vi "load_xml_2.vi"(8 "error in":errorcluster, 10 "child node in":refnum<k20>, 11 "HSDIO (in)":refnum<class "HSDIO.lvclass">) -> (0 "error out":errorcluster, 2 "child node out":refnum<k20>, 3 "HSDIO":refnum<class "HSDIO.lvclass">)   [LabVIEW 2013, in "HSDIO.lvclass"]
doc: "Loads HSDIO settings from xml. Expected format:\n\n<EnableHSDIOPulses>%b</EnableHSDIOPulses>\n<ResourceName>%s</ResourceName>\n<ClockRate>%f</ClockRate>\n<unitsPerSecond>%f</unitsPerSecond>\n<HardwareAlignmentQuantum units=\"samples\">%u</HardwareAlignmentQuantum>\n<ArrayOfScriptTriggers columns=\"id, source, type, edge, level\">\n<trigger>%s\\t%s\\t%s\\t%s\\t%s</trigger>\n</ArrayOfScriptTriggers>\n<ChannelsControl columns=\"Description, Active?, Idle State\">\n<channel>%s</channel>\n</ChannelsControl>\n<PulseGenerationScript>%s</PulseGenerationScript>\n<DirectoryToLookForWaveformFiles>%s</DirectoryToLookForWaveformFiles>\n<StartTrigger.WaitForStartTrigger>%b</StartTrigger.WaitForStartTrigger>\n<StartTrigger.source>%s</StartTrigger.source>\n<StartTrigger.edge>%s</StartTrigger.edge>\n\nMTL 2013 Jan 1"
uses:
  HSDIO.lvclass
  HSDIO.lvclass/HSDIO.ctl
  <instrlib>/niHSDIO/niHSDIO.llb/niHSDIO_ctl Trigger Script - trigID Values (Ring).ctl
  <instrlib>/niHSDIO/niHSDIO.llb/niHSDIO_ctl Trigger Source Values (Ring).ctl
  <instrlib>/niHSDIO/niHSDIO.llb/niHSDIO_ctl Trigger DigEdge - Edge Values (Ring).ctl
  <instrlib>/niHSDIO/niHSDIO.llb/niHSDIO_ctl Trigger DigLvl - Level Values (Ring).ctl
  waveform.ctl
  <vilib>/xml/Close Reference(Node).vi
  <resource>/objmgr/DOMUserDefRef.rc
  <vilib>/xml/NI_XML.lvlib
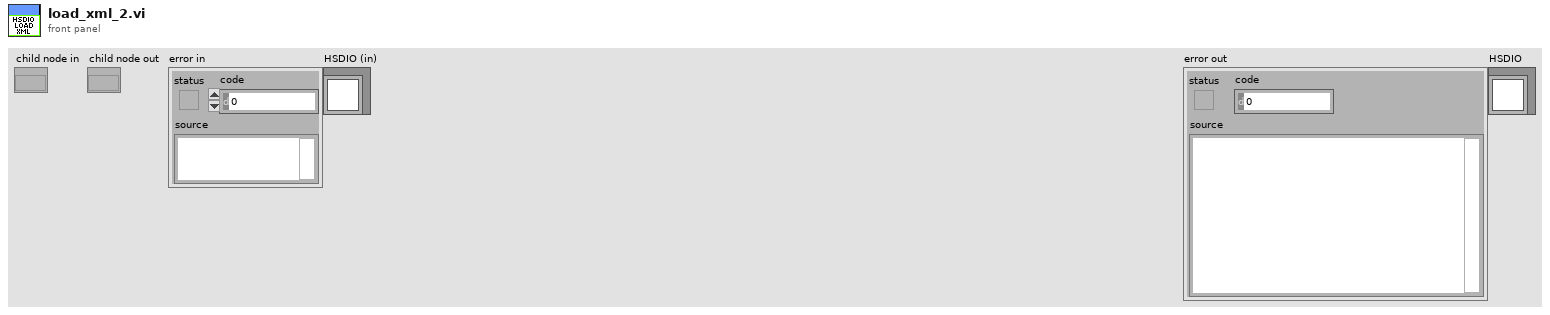
[diagram p1: front panel]
types:
  T1 = typedef "niHSDIO_ctl Trigger Script - trigID Values (Ring).ctl" = string
  T2 = typedef "niHSDIO_ctl Trigger Source Values (Ring).ctl" = string
  T3 = typedef "niHSDIO_ctl Trigger DigEdge - Edge Values (Ring).ctl" = i32
  T4 = typedef "niHSDIO_ctl Trigger DigLvl - Level Values (Ring).ctl" = i32
  T5 = cluster{"trigger id (script trigger 0)":T1, "source (PFI 0)":T2, "Trigger Type":enum32{"Edge", "Level"}, "edge":T3, "level":T4}
  T6 = typedef "HSDIO.lvclass/HSDIO_settings.ctl" = cluster{"Enable HSDIO Pulses":bool, "Resource Name":refnum<k15>, "Clock Rate":dbl, "units/sec (ms=1000)":dbl, "Array of Script Triggers":cluster{"trigger id (script trigger 0)":T1, "source (PFI 0)":T2, "Trigger Type":enum32{"Edge", "Level"}, "edge":T3, "level":T4}[], "Channels Control":string[][], "Pulse Generation Script":string, "Directory to look for waveform files":path, "Start Trigger":cluster{"Wait for start trigger?":bool, "source (PFI 0)":T2, "edge (rising)":T3}, "Hardware alignment quantum\n(in samples)":u16, "Use file script":bool, "Base path for script":path, "filename for script":string, "Inital State":string, "Idle State":string, "Active Channels":string, "Array of Waveforms":T7[]}
  T7 = typedef "HSDIO.lvclass/waveform.ctl" = cluster{"name":string, "transitions":u32[], "states":u8[][]}
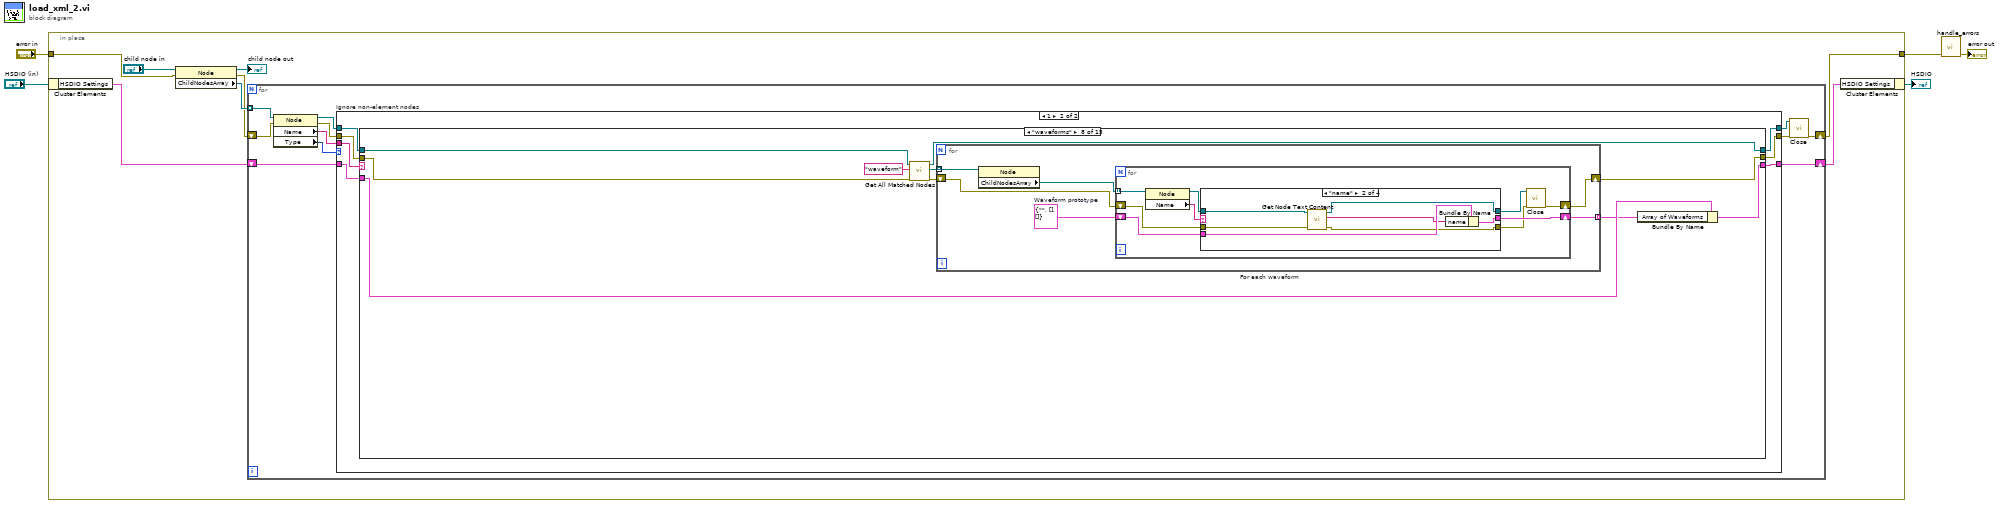
[diagram p0: block diagram]
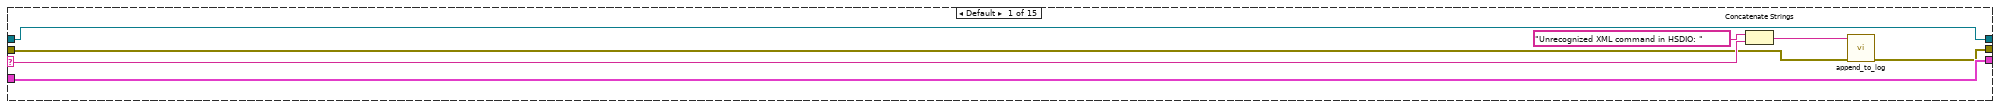
[diagram p3: hidden frame]
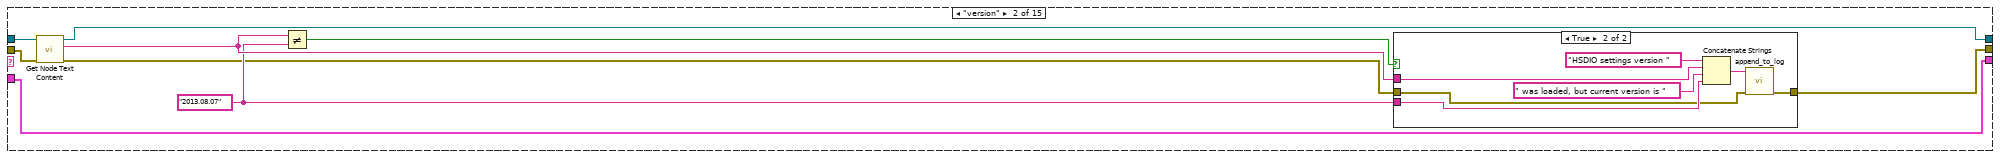
[diagram p4: hidden frame]
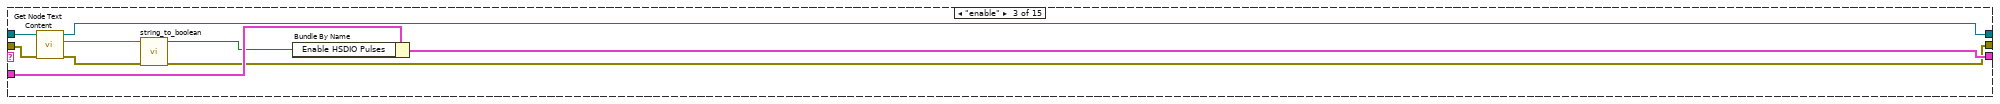
[diagram p6: hidden frame]
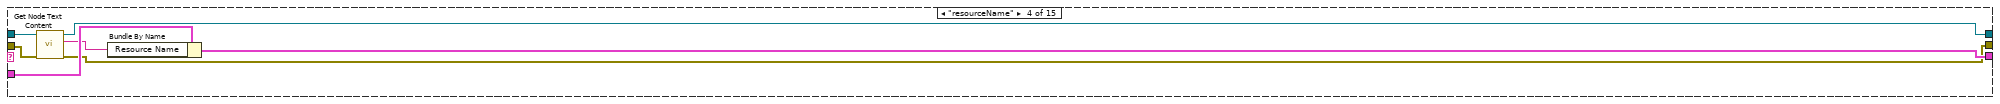
[diagram p7: hidden frame]
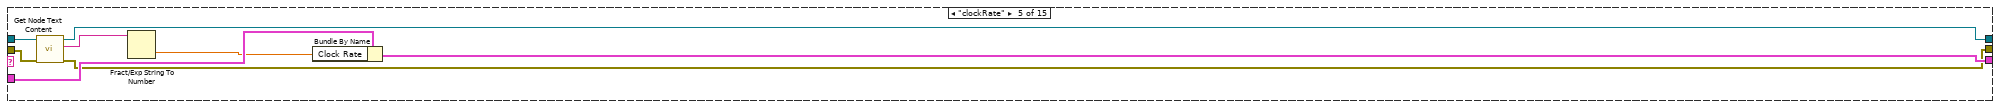
[diagram p8: hidden frame]
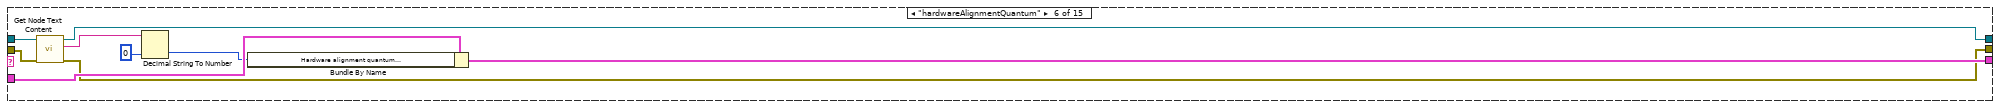
[diagram p9: hidden frame]
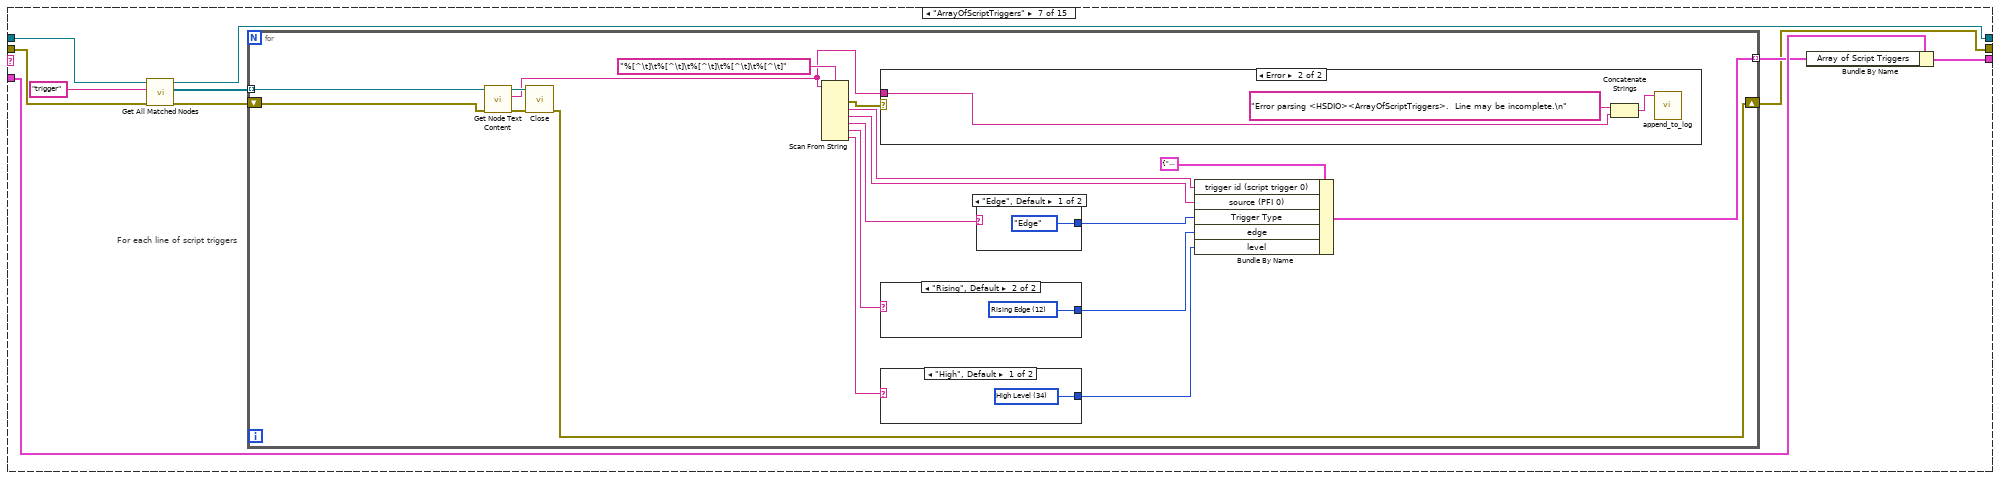
[diagram p10: hidden frame]
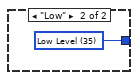
[diagram p11: hidden frame]
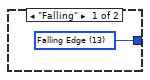
[diagram p12: hidden frame]
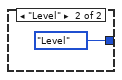
[diagram p13: hidden frame]
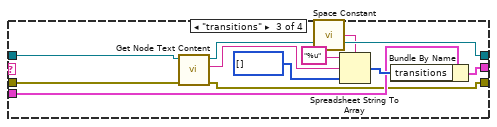
[diagram p16: hidden frame]
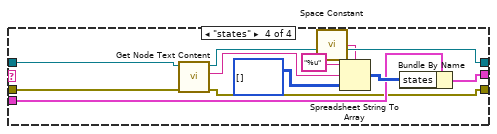
[diagram p17: hidden frame]
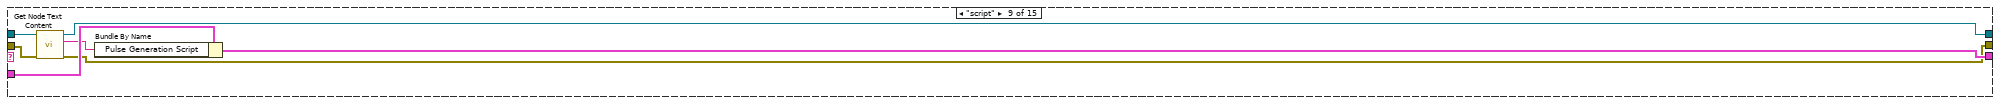
[diagram p18: hidden frame]
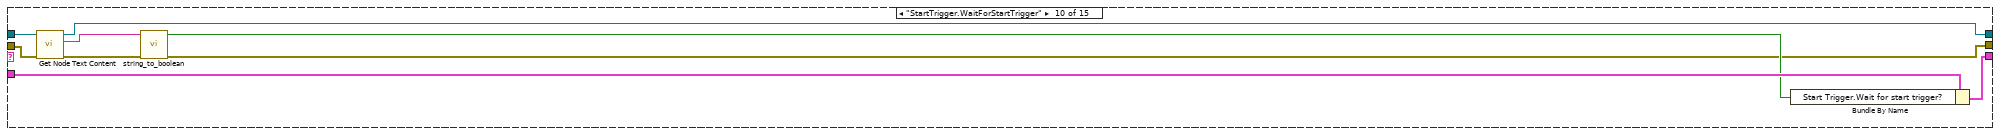
[diagram p19: hidden frame]
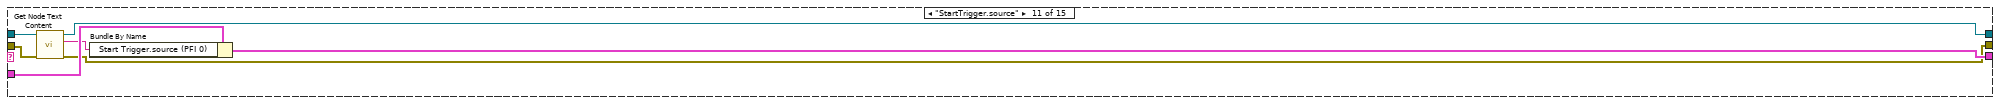
[diagram p20: hidden frame]
diagram:
  n1 = in-place {
    in-place-border: "error in" -> [w9]
    in-place-border: [w7] -> w2
    n2 = in-place-cluster #1("HSDIO (in)") -> ("HSDIO Settings"=w6:T6)
    n3 = property class="Node"(reference="child node in", error in=w9) -> (reference out=→"child node out":refnum<k20>, error out=w11:errorcluster, "ChildNodesArray"=w13:refnum<k20>[])
    n4 = for {
      tunnel: w13 -> [w19] mode=indexing
      shift-right: [w21] -> w8
      shift-left: w6 -> [w22]
      shift-right: [w15] -> w7
      shift-left: w11 -> [w18]
      n5 = property class="Node"(reference=w19, error in=w18) -> (reference out=w23:refnum<k20>, error out=w20:errorcluster, "Name"=w24:string, "Type"=w17:i32)
      n6 = case "Ignore non-element nodes" shown="1" w17 {
        tunnel: w24 -> [_ w34]
        tunnel: w23 -> [w25 w33]
        tunnel: w22 -> [w26 w32]
        tunnel: [w26 w31] -> w21
        tunnel: w20 -> [w27 w30]
        tunnel: [w27 w29] -> w16
        tunnel: [w25 w28] -> w14
        frame Default {
        }
        frame 1 {
          n7 = case shown="\"waveforms\"" w34 {
            selector: w34 -> [w37 _ _ _ _ _ _ _ _ _ _ _ _ _ _]
            tunnel: w33 -> [w40 w46 w66 w71 w79 w87 w101 w138 w189 w200 w205 w213 w222 w229 w236]
            tunnel: w32 -> [w41 w44 w64 w74 w82 w91 w98 w135 w192 w198 w208 w216 w225 w232 w239]
            tunnel: [w41 w44 w63 w73 w81 w90 w96 w133 w191 w197 w207 w215 w224 w231 w238] -> w31
            tunnel: [w40 w43 w67 w72 w80 w86 w95 w132 w190 w201 w206 w214 w223 w230 w237] -> w28
            tunnel: w30 -> [w36 w45 w65 w70 w78 w85 w94 w131 w188 w199 w204 w212 w221 w228 w235]
            tunnel: [w35 w42 w59 w69 w77 w84 w92 w129 w187 w193 w203 w211 w220 w227 w234] -> w29
            frame Default {
              n8 = Concatenate Strings("Unrecognized XML command in HSDIO: " ("string"), w37) -> (w38:string)
              n9 = call "append_to_log.vi"("error in"=w36, "string"=w38) -> ("error out"=w35:errorcluster)  [unwired: 9 in]
            }
            frame "version" {
              w48 = "2013.08.07" ("y")
              n10 = call <vilib>:"Get Node Text Content.vi"("error in (no error)"=w45, "node in"=w46) -> ("error out"=w47:errorcluster, "node text"=w49:string, "node out"=w43:refnum<k20>)  [unwired: 7 in]
              n11 = Not Equal?(x=w49, y=w48) -> (x != y?=w50:bool)
              n12 = case shown="True" w50 {
                tunnel: w49 -> [_ w57]
                tunnel: w48 -> [_ w55]
                tunnel: w47 -> [w51 w53]
                tunnel: [w51 w52] -> w42
                frame False {
                }
                frame True {
                  n13 = Concatenate Strings("HSDIO settings version " ("string"), w57, " was loaded, but current version is " ("string"), w55) -> (w54:string)
                  n14 = call "append_to_log.vi"("error in"=w53, "string"=w54) -> ("error out"=w52:errorcluster)  [unwired: 9 in]
                }
              }
            }
            frame "enable" {
              n15 = call <vilib>:"Get Node Text Content.vi"("error in (no error)"=w65, "node in"=w66) -> ("error out"=w60:errorcluster, "node text"=w62:string, "node out"=w67:refnum<k20>)  [unwired: 7 in]
              n16 = call "string_to_boolean.vi"("error in"=w60, "string"=w62) -> ("error out"=w59:errorcluster, "boolean"=w61:bool)  [unwired: 8 in]
              n17 = Bundle By Name(cluster=w64, "Enable HSDIO Pulses"=w61) -> (w63:T6)
            }
            frame "resourceName" {
              n18 = call <vilib>:"Get Node Text Content.vi"("error in (no error)"=w70, "node in"=w71) -> ("error out"=w69:errorcluster, "node text"=w68:string, "node out"=w72:refnum<k20>)  [unwired: 7 in]
              n19 = Bundle By Name(cluster=w74, "Resource Name"=w68) -> (w73:T6)
            }
            frame "clockRate" {
              n20 = call <vilib>:"Get Node Text Content.vi"("error in (no error)"=w78, "node in"=w79) -> ("error out"=w77:errorcluster, "node text"=w76:string, "node out"=w80:refnum<k20>)  [unwired: 7 in]
              n21 = Fract/Exp String To Number(string=w76) -> (number=w75:dbl)  [unwired: 3 in, 1 out]
              n22 = Bundle By Name(cluster=w82, "Clock Rate"=w75) -> (w81:T6)
            }
            frame "hardwareAlignmentQuantum" {
              n23 = call <vilib>:"Get Node Text Content.vi"("error in (no error)"=w85, "node in"=w87) -> ("error out"=w84:errorcluster, "node text"=w89:string, "node out"=w86:refnum<k20>)  [unwired: 7 in]
              n24 = Decimal String To Number(string=w89, default (0L)=u16 0 ("default (0 I32)")) -> (number=w88:u16)  [unwired: 1 in, 1 out]
              n25 = Bundle By Name(cluster=w91, "Hardware alignment quantum\n(in samples)"=w88) -> (w90:T6)
            }
            frame "ArrayOfScriptTriggers" {
              n26 = call <vilib>:"Get All Matched Nodes.vi"("error in (no error)"=w94, "XPath expression"="trigger", "node in"=w101) -> ("error out"=w93:errorcluster, "node result array"=w99:refnum<k20>[], "node out"=w95:refnum<k20>)  [unwired: 6 in]
              n27 = for "For each line of script triggers" {
                tunnel: w99 -> [w117] mode=indexing
                tunnel: [w118] -> w97 mode=indexing
                shift-right: [w114] -> w92
                shift-left: w93 -> [w115]
                n28 = call <vilib>:"Get Node Text Content.vi"("error in (no error)"=w115, "node in"=w117) -> ("error out"=w106:errorcluster, "node text"=w102:string, "node out"=w116:refnum<k20>)  [unwired: 7 in]
                n29 = call-poly <vilib>:"Close.vi"("error in (no error)"=w106, "node"=w116) -> ("error out"=w114:errorcluster)  [unwired: 7 in]
                n30 = Scan From String(format string="%[^\t]\t%[^\t]\t%[^\t]\t%[^\t]\t%[^\t]", input string=w102) -> (error out=w103:errorcluster, output 1=w105:string, output 2=w104:string, output 3=w113:string, output 4=w111:string, output 5=w109:string)  [unwired: 7 in, 2 out]
                n31 = case shown="Error" w103 {
                  tunnel: w102 -> [_ w126]
                  frame No Error {
                  }
                  frame Error {
                    n32 = Concatenate Strings("Error parsing <HSDIO><ArrayOfScriptTriggers>.  Line may be incomplete.\n" ("string"), w126) -> (w127:string)
                    n33 = call "append_to_log.vi"("string"=w127) -> ()  [unwired: 10 in, 1 out]
                  }
                }
                n34 = case shown="\"Rising\", Default" w111 {
                  tunnel: [w122 w123] -> w110
                  frame "Falling" {
                    w122 = T3 13 items=["Rising Edge"=12, "Falling Edge"=13] ("edge")
                  }
                  frame "Rising", Default {
                    w123 = T3 12 items=["Rising Edge"=12, "Falling Edge"=13] ("edge")
                  }
                }
                n35 = case shown="\"High\", Default" w109 {
                  tunnel: [w120 w121] -> w108
                  frame "High", Default {
                    w120 = T4 34 items=["High Level"=34, "Low Level"=35] ("level")
                  }
                  frame "Low" {
                    w121 = T4 35 items=["High Level"=34, "Low Level"=35] ("level")
                  }
                }
                n36 = case shown="\"Edge\", Default" w113 {
                  tunnel: [enum32{"Edge", "Level"}."Edge" ("Trigger Type") enum32{"Edge", "Level"}."Level" ("Trigger Type")] -> w112
                  frame "Edge", Default {
                  }
                  frame "Level" {
                  }
                }
                n37 = Bundle By Name(cluster=T5 {"trigger id (script trigger 0)"="", "source (PFI 0)"="", "Trigger Type"=enum."Edge", "edge"=0, "level"=0} ("Script Trigger"), "trigger id (script trigger 0)"=w105, "source (PFI 0)"=w104, "Trigger Type"=w112, "edge"=w110, "level"=w108) -> (w118:T5)
              }
              n38 = Bundle By Name(cluster=w98, "Array of Script Triggers"=w97) -> (w96:T6)
            }
            frame "waveforms" {
              n39 = call <vilib>:"Get All Matched Nodes.vi"("error in (no error)"=w131, "XPath expression"="waveform", "node in"=w138) -> ("error out"=w130:errorcluster, "node result array"=w136:refnum<k20>[], "node out"=w132:refnum<k20>)  [unwired: 6 in]
              n40 = for "For each waveform" {
                tunnel: w136 -> [w144] mode=indexing
                tunnel: [w141] -> w134 mode=indexing
                shift-right: [w139] -> w129
                shift-left: w130 -> [w140]
                w142 = T7 {"name"="", "transitions"=[], "states"=[]}  # Waveform prototype
                n41 = property class="Node"(reference=w144) -> ("ChildNodesArray"=w143:refnum<k20>[])  [unwired: 1 in, 2 out]
                n42 = for {
                  tunnel: w143 -> [w153] mode=indexing
                  shift-right: [w150] -> w141
                  shift-left: w142 -> [w151]
                  shift-right: [w145] -> w139
                  shift-left: w140 -> [w147]
                  n43 = property class="Node"(reference=w153) -> (reference out=w149:refnum<k20>, "Name"=w152:string)  [unwired: 1 in, 1 out]
                  n44 = case shown="\"name\"" w152 {
                    tunnel: w151 -> [w155 w163 w170 w181]
                    tunnel: [w155 w162 w169 w180] -> w150
                    tunnel: w149 -> [w156 w161 w167 w178]
                    tunnel: [w156 w160 w168 w179] -> w148
                    tunnel: w147 -> [w154 w159 w166 w177]
                    tunnel: [w154 w157 w165 w176] -> w146
                    frame Default {
                    }
                    frame "name" {
                      n45 = call <vilib>:"Get Node Text Content.vi"("error in (no error)"=w159, "node in"=w161) -> ("error out"=w157:errorcluster, "node text"=w158:string, "node out"=w160:refnum<k20>)  [unwired: 7 in]
                      n46 = Bundle By Name(cluster=w163, "name"=w158) -> (w162:T7)
                    }
                    frame "transitions" {
                      n47 = call <vilib>:"Get Node Text Content.vi"("error in (no error)"=w166, "node in"=w167) -> ("error out"=w165:errorcluster, "node text"=w172:string, "node out"=w168:refnum<k20>)  [unwired: 7 in]
                      n48 = call <vilib>:"Space Constant.vi"() -> ("String"=w164:string)
                      n49 = Spreadsheet String To Array(delimiter (Tab)=w164, format string="%u", spreadsheet string=w172, array type (2D Dbl)=u32[] []) -> (array=w171:u32[])
                      n50 = Bundle By Name(cluster=w170, "transitions"=w171) -> (w169:T7)
                    }
                    frame "states" {
                      n51 = call <vilib>:"Get Node Text Content.vi"("error in (no error)"=w177, "node in"=w178) -> ("error out"=w176:errorcluster, "node text"=w183:string, "node out"=w179:refnum<k20>)  [unwired: 7 in]
                      n52 = call <vilib>:"Space Constant.vi"() -> ("String"=w175:string)
                      n53 = Spreadsheet String To Array(delimiter (Tab)=w175, format string="%u", spreadsheet string=w183, array type (2D Dbl)=u8[][] []) -> (array=w182:u8[][])
                      n54 = Bundle By Name(cluster=w181, "states"=w182) -> (w180:T7)
                    }
                  }
                  n55 = call-poly <vilib>:"Close.vi"("error in (no error)"=w146, "node"=w148) -> ("error out"=w145:errorcluster)  [unwired: 7 in]
                }
              }
              n56 = Bundle By Name(cluster=w135, "Array of Waveforms"=w134) -> (w133:T6)
            }
            frame "script" {
              n57 = call <vilib>:"Get Node Text Content.vi"("error in (no error)"=w188, "node in"=w189) -> ("error out"=w187:errorcluster, "node text"=w186:string, "node out"=w190:refnum<k20>)  [unwired: 7 in]
              n58 = Bundle By Name(cluster=w192, "Pulse Generation Script"=w186) -> (w191:T6)
            }
            frame "StartTrigger.WaitForStartTrigger" {
              n59 = call <vilib>:"Get Node Text Content.vi"("error in (no error)"=w199, "node in"=w200) -> ("error out"=w194:errorcluster, "node text"=w196:string, "node out"=w201:refnum<k20>)  [unwired: 7 in]
              n60 = call "string_to_boolean.vi"("error in"=w194, "string"=w196) -> ("error out"=w193:errorcluster, "boolean"=w195:bool)  [unwired: 8 in]
              n61 = Bundle By Name(cluster=w198, "Start Trigger.Wait for start trigger?"=w195) -> (w197:T6)
            }
            frame "StartTrigger.source" {
              n62 = call <vilib>:"Get Node Text Content.vi"("error in (no error)"=w204, "node in"=w205) -> ("error out"=w203:errorcluster, "node text"=w202:string, "node out"=w206:refnum<k20>)  [unwired: 7 in]
              n63 = Bundle By Name(cluster=w208, "Start Trigger.source (PFI 0)"=w202) -> (w207:T6)
            }
            frame "StartTrigger.edge" {
              n64 = call <vilib>:"Get Node Text Content.vi"("error in (no error)"=w212, "node in"=w213) -> ("error out"=w211:errorcluster, "node text"=w210:string, "node out"=w214:refnum<k20>)  [unwired: 7 in]
              n65 = case "Convert Enum to string" shown="\"Falling\"" w210 {
                tunnel: [w217 w218] -> w209
                frame "Falling" {
                  w217 = T3 13 items=["Rising Edge"=12, "Falling Edge"=13] ("Start Trigger.edge (rising)")
                }
                frame "Rising", Default {
                  w218 = T3 12 items=["Rising Edge"=12, "Falling Edge"=13] ("Start Trigger.edge (rising)")
                }
              }
              n66 = Bundle By Name(cluster=w216, "Start Trigger.edge (rising)"=w209) -> (w215:T6)
            }
            frame "InitialState" {
              n67 = call <vilib>:"Get Node Text Content.vi"("error in (no error)"=w221, "node in"=w222) -> ("error out"=w220:errorcluster, "node text"=w219:string, "node out"=w223:refnum<k20>)  [unwired: 7 in]
              n68 = Bundle By Name(cluster=w225, "Inital State"=w219) -> (w224:T6)
            }
            frame "IdleState" {
              n69 = call <vilib>:"Get Node Text Content.vi"("error in (no error)"=w228, "node in"=w229) -> ("error out"=w227:errorcluster, "node text"=w226:string, "node out"=w230:refnum<k20>)  [unwired: 7 in]
              n70 = Bundle By Name(cluster=w232, "Idle State"=w226) -> (w231:T6)
            }
            frame "ActiveChannels" {
              n71 = call <vilib>:"Get Node Text Content.vi"("error in (no error)"=w235, "node in"=w236) -> ("error out"=w234:errorcluster, "node text"=w233:string, "node out"=w237:refnum<k20>)  [unwired: 7 in]
              n72 = Bundle By Name(cluster=w239, "Active Channels"=w233) -> (w238:T6)
            }
          }
        }
      }
      n73 = call-poly <vilib>:"Close.vi"("error in (no error)"=w16, "node"=w14) -> ("error out"=w15:errorcluster)  [unwired: 7 in]
    }
    n74 = in-place-cluster #1("HSDIO Settings"=w8) -> (→"HSDIO":refnum<class "HSDIO.lvclass">)
  }
  n75 = call "handle_errors.vi"("error in (no error)"=w2) -> ("error out"=→"error out":errorcluster)  [unwired: 10 in]
